vi "Multicolumn Edit Cells.vi"(8 "error in (no error)":errorcluster, 11 "ZenGage v3.0 UI in":refnum<class "ZenGage v3.0 UI.lvclass">) -> (0 "error out":errorcluster, 3 "ZenGage v3.0 UI out":refnum<class "ZenGage v3.0 UI.lvclass">)   [LabVIEW 2015, in "ZenGage v3.0 UI.lvclass"]
uses:
  ZenGage v3.0 UI.lvclass
  <vilib>/Utility/miscctls.llb/LVRowAndColumnTypeDef.ctl
  ZenGage v3.0 UI.lvclass/ZenGage v3.0 UI.ctl
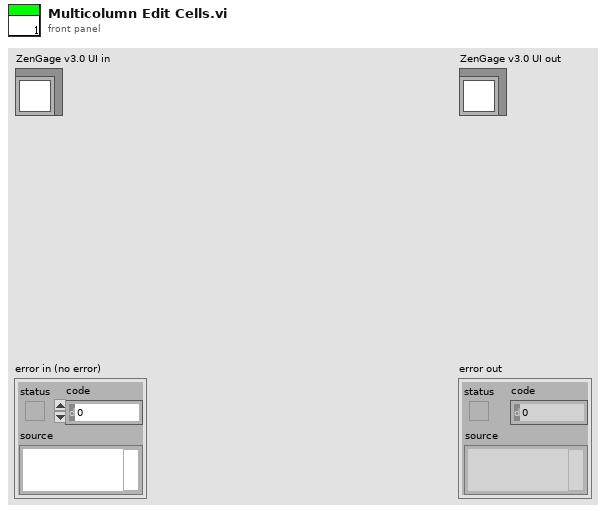
[diagram p1: front panel]
types:
  T1 = typedef "LVRowAndColumnTypeDef.ctl" = cluster{"Row":i32, "Column":i32}
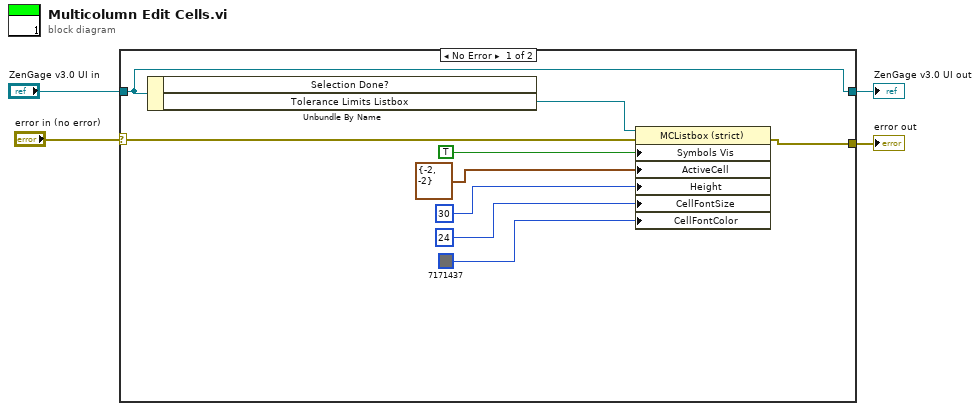
[diagram p0: block diagram]
diagram:
  n1 = case shown="No Error" "error in (no error)" {
    selector: "error in (no error)" -> [w6 w15]
    tunnel: [w5 w15] -> w3
    tunnel: [w13 w14] -> w1
    tunnel: "ZenGage v3.0 UI in" -> [w13 w14]
    frame No Error {
      n2 = Unbundle By Name(w13) -> ("Tolerance Limits Listbox"=w7:refnum<vi>)  [unwired: 1 out]
      n3 = property class="MCListbox (strict)"(reference=w7, error in=w6, "Symbols Vis"=TRUE ("Visible Items:Symbols Visible"), "ActiveCell"=T1 {"Row"=-2, "Column"=-2} ("Active Cell:Active Cell"), "Height"=u32 30 ("Active Cell:Cell Size:Height"), "CellFontSize"=u32 24 ("Active Cell:Cell Font:Size"), "CellFontColor"=u32 7171437) -> (error out=w5:errorcluster)  [unwired: 1 out]
    }
    frame Error {
    }
  }
  "error out" <- w3
  "ZenGage v3.0 UI out" <- w1
